vi "Couple Hex to ASCII.vi"(6 "HEX_LB In":string[](array[string]), 7 "HEX_UB In":string[](array[string]), 8 "error in (no error)":errorcluster) -> (0 "Error Out":errorcluster, 1 "HEX_UB":string[](array[string]), 3 "HEX_LB":string[](array[string]), 4 "ASCII_LB":string[](array[string]), 5 "ASCII_UB":string[](array[string]))   [LabVIEW 2017]
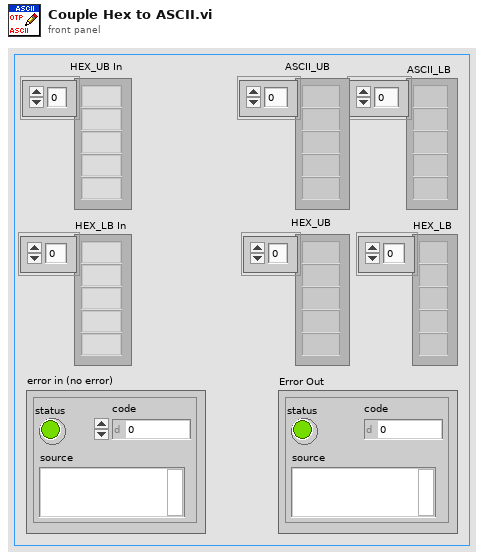
[diagram p1: front panel]
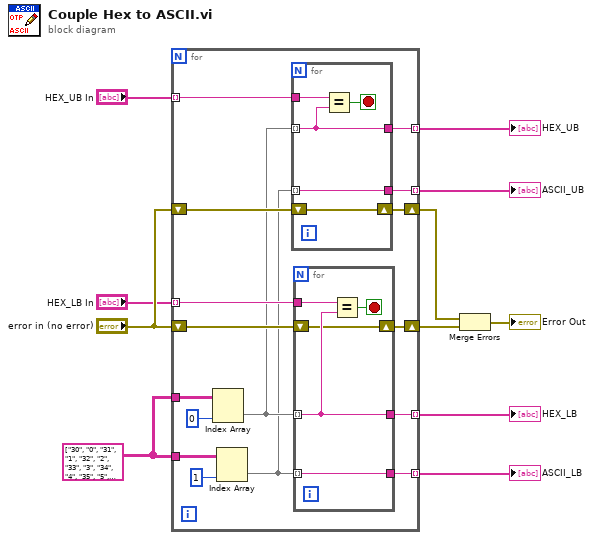
[diagram p0: block diagram]
diagram:
  w11 = string[][] [["30", "0"], ["31", "1"], ["32", "2"], ["33", "3"], ["34", "4"], ["35", "5"], ["36", "6"], ["37", "7"], ["38", "8"], ["39", "9"], ["41", "A"], ["42", "B"], ["43", "C"], ["44", "D"], ["45", "E"], ["46", "F"], ["47", "G"], ["48", "H"], ["49", "I"], ["4A", "J"], ["4B", "K"], ["4C", "L"], ["4D", "M"], ["4E", "N"], ["4F", "O"], ["50", "P"], ["51", "Q"], ["52", "R"], ["53", "S"], ["54", "T"], ["55", "U"], ["56", "V"], ["57", "W"], ["58", "X"], ["59", "Y"], ["5A", "Z"], ["61", "a"], ["62", "b"], ["63", "c"], ["64", "d"], ["65", "e"], ["66", "f"], ["67", "g"], ["68", "h"], ["69", "i"], ["6A", "j"], ["6B", "k"], ["6C", "l"], ["6D", "m"], ["6E", "n"], ["6F", "o"], ["70", "p"], ["71", "q"], ["72", "r"], ["73", "s"], ["74", "t"], ["75", "u"], ["76", "v"], ["77", "w"], ["78", "x"], ["79", "y"], ["7A", "z"]] ("all rows")
  n1 = for {
    tunnel: "HEX_LB In" -> [w23] mode=indexing
    tunnel: w11 -> [w27]
    tunnel: w11 -> [w26]
    tunnel: [w22] -> w2 mode=indexing
    tunnel: [w21] -> w1 mode=indexing
    shift-right: [w20] -> w10
    shift-left: "error in (no error)" -> [w19]
    shift-right: [w18] -> w9
    shift-left: "error in (no error)" -> [w17]
    tunnel: "HEX_UB In" -> [w16] mode=indexing
    tunnel: [w13] -> w4 mode=indexing
    tunnel: [w12] -> w3 mode=indexing
    n2 = Index Array(array=w27, index (col)=0 ("index")) -> (element=w15:string[])  [unwired: 1 in]
    n3 = Index Array(array=w26, index (col)=1 ("index")) -> (element=w14:string[])  [unwired: 1 in]
    n4 = for {
      shift-right: [w32] -> w18
      shift-left: w17 -> [w32]
      tunnel: w16 -> [w31]
      tunnel: w15 -> [w29] mode=indexing
      tunnel: w14 -> [w30] mode=indexing
      tunnel: [w30] -> w13
      tunnel: [w29] -> w12
      stop <- w28 stop-if-true
      n5 = Equal?(x=w31, y=w29) -> (x = y?=w28:bool)
    }
    n6 = for {
      tunnel: w23 -> [w37]
      tunnel: w15 -> [w35] mode=indexing
      tunnel: w14 -> [w34] mode=indexing
      tunnel: [w35] -> w22
      tunnel: [w34] -> w21
      shift-right: [w33] -> w20
      shift-left: w19 -> [w33]
      stop <- w36 stop-if-true
      n7 = Equal?(x=w37, y=w35) -> (x = y?=w36:bool)
    }
  }
  "ASCII_LB" <- w1
  "HEX_LB" <- w2
  "ASCII_UB" <- w4
  "HEX_UB" <- w3
  n8 = Merge Errors(w9, w10) -> (→"Error Out":errorcluster)
